vi "SaveIMAQImage.vi"(8 "error in (no error)":errorcluster, 10 "Path":path, 11 "Photometrics Cam v2 in":refnum<class "Photometrics_CH-250_Cam.lvclass">) -> (0 "error out":errorcluster, 3 "Photometrics Cam v2out":refnum<class "Photometrics_CH-250_Cam.lvclass">)   [LabVIEW 2013, in "Photometrics_CH-250_Cam.lvclass"]
uses:
  Photometrics_CH-250_Cam.lvclass
  Photometrics_CH-250_Cam.lvclass/Photometrics_CH-250_Cam.ctl
  CameraSessionClass/CS250-CameraHardwareClass.lvclass
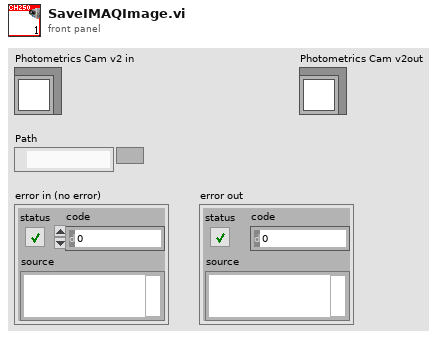
[diagram p1: front panel]
types:
  T1 = typedef "IMAQ Image.ctl" = refnum<image>
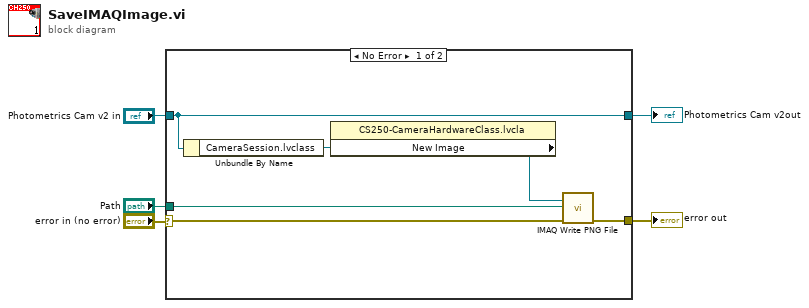
[diagram p0: block diagram]
diagram:
  n1 = case shown="No Error" "error in (no error)" {
    selector: "error in (no error)" -> [w7 w12]
    tunnel: [w9 w12] -> w5
    tunnel: "Path" -> [w8 _]
    tunnel: "Photometrics Cam v2 in" -> [w6 w13]
    tunnel: [w6 w13] -> w1
    frame No Error {
      n2 = Unbundle By Name(w6) -> ("CameraSession.lvclass"=w10:refnum<class "CS250-CameraHardwareClass.lvclass">)
      n3 = property class="CS250-CameraHardwareClass.lvcla"(reference=w10) -> ("New Image"=w11:T1)  [unwired: 1 in, 2 out]
      n4 = call "IMAQ Write PNG File"("error in (no error)"=w7, "File Path"=w8, "Image"=w11) -> ("error out"=w9:errorcluster)  [unwired: 3 in, 2 out]
    }
    frame Error {
    }
  }
  "error out" <- w5
  "Photometrics Cam v2out" <- w1
